vi "Shift State.vi"(6 "Lower bound":i32, 7 "Upper bound":i32, 9 "Decrement":bool, 10 "Increment":bool, 11 "State in":i32) -> (3 "State out":i32)   [LabVIEW 2014]
doc: "Shifts a state up or down by 1.\nUsed in the operation of the elevator, clapper, and arm angle."
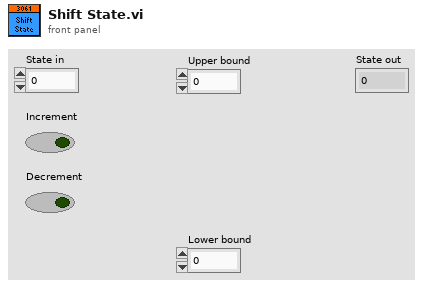
[diagram p1: front panel]
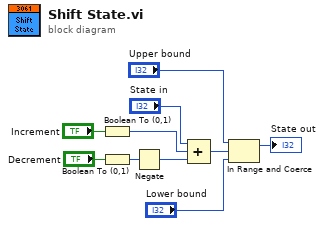
[diagram p0: block diagram]
diagram:
  n1 = Boolean To (0,1)(Boolean="Increment") -> (0, 1=w3:i16)
  n2 = Boolean To (0,1)(Boolean="Decrement") -> (0, 1=w8:i16)
  n3 = Negate(x=w8) -> (-x=w2:i16)
  n4 = Compound Arithmetic op=ADD("State in", w3, w2) -> (w1:i32)
  n5 = In Range and Coerce(upper limit="Upper bound", x=w1, lower limit="Lower bound") -> (coerced(x)=→"State out":i32)  [unwired: 1 out]
